vi "Delete me.vi"(10 "Debug":bool, 11 "State Pts in":T1) -> (2 "output cluster":cluster{dbl[], dbl[]}, 3 "State Pts out":T1)   [LabVIEW 2012]
uses:
  STARCO-Dev/RT-PID/support/P-h Diagram/States In.ctl
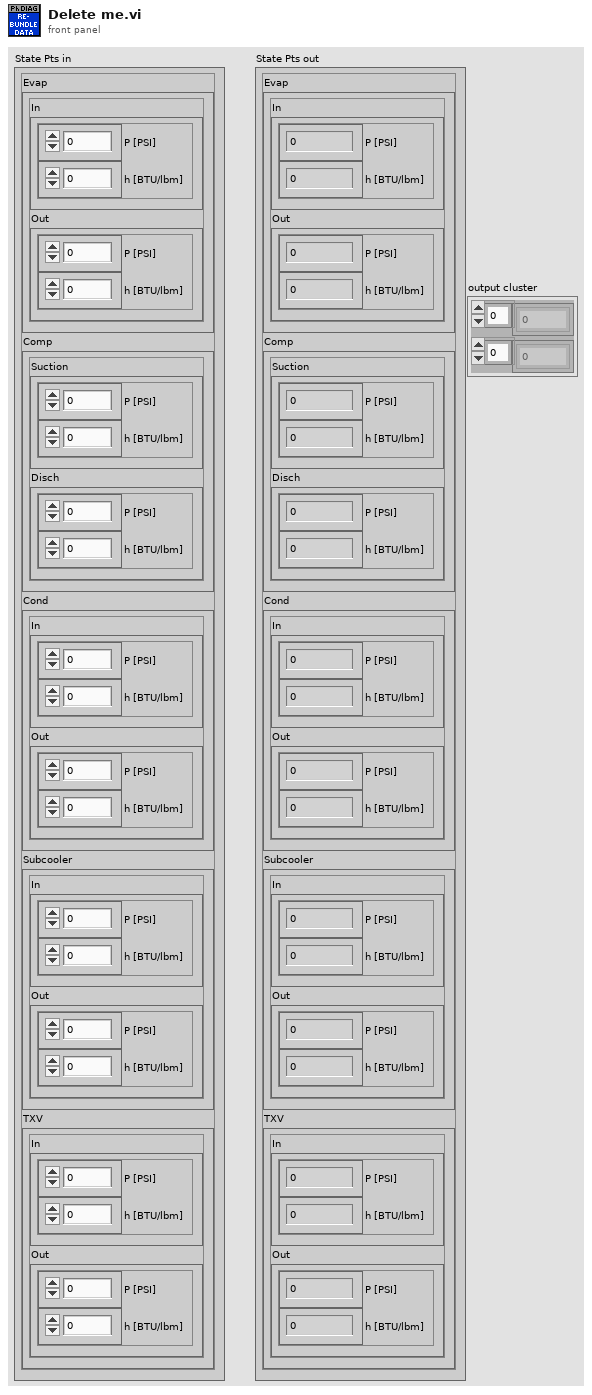
[diagram p1: front panel]
types:
  T1 = typedef "States In.ctl" = cluster{"Evap":cluster{"In":cluster{"P [PSI]":dbl, "h [BTU/lbm]":dbl}, "Out":cluster{"P [PSI]":dbl, "h [BTU/lbm]":dbl}}, "Comp":cluster{"Suction":cluster{"P [PSI]":dbl, "h [BTU/lbm]":dbl}, "Disch":cluster{"P [PSI]":dbl, "h [BTU/lbm]":dbl}}, "Cond":cluster{"In":cluster{"P [PSI]":dbl, "h [BTU/lbm]":dbl}, "Out":cluster{"P [PSI]":dbl, "h [BTU/lbm]":dbl}}, "Subcooler":cluster{"In":cluster{"P [PSI]":dbl, "h [BTU/lbm]":dbl}, "Out":cluster{"P [PSI]":dbl, "h [BTU/lbm]":dbl}}, "TXV":cluster{"In":cluster{"P [PSI]":dbl, "h [BTU/lbm]":dbl}, "Out":cluster{"P [PSI]":dbl, "h [BTU/lbm]":dbl}}}
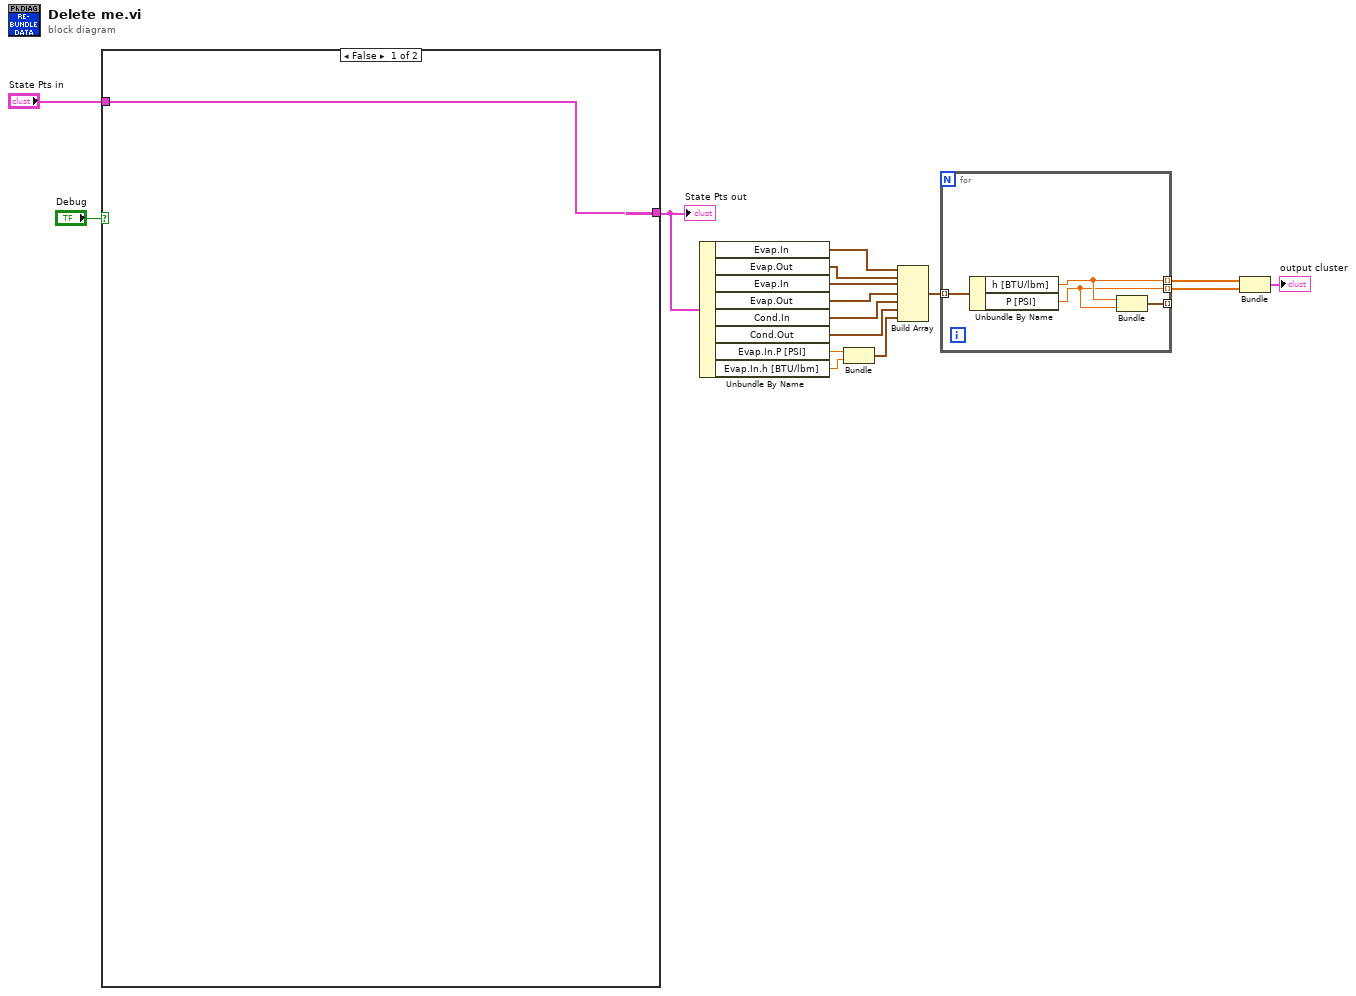
[diagram p0: block diagram]
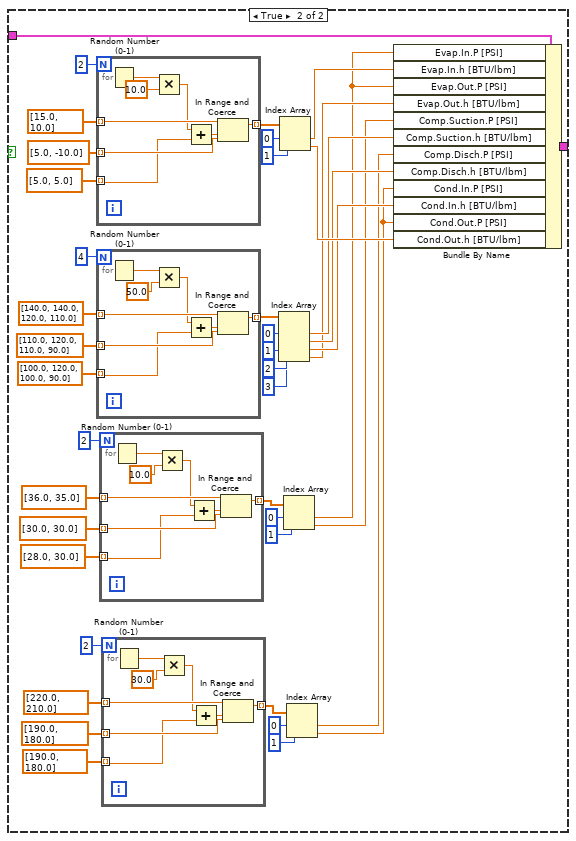
[diagram p2: hidden frame]
diagram:
  n1 = case shown="False" "Debug" {
    tunnel: "State Pts in" -> [w17 w59]
    tunnel: [w17 w58] -> w4
    frame False {
    }
    frame True {
      n2 = for {
        N: 2 -> [_]
        tunnel: dbl[] [15.0, 10.0] -> [w89] mode=indexing
        tunnel: dbl[] [5.0, -10.0] -> [w88] mode=indexing
        tunnel: dbl[] [5.0, 5.0] -> [w86] mode=indexing
        tunnel: [w85] -> w45 mode=indexing
        n3 = Random Number (0-1)() -> (number: 0 to 1=w90:dbl)
        n4 = Multiply(x=w90, y=10.0) -> (x*y=w87:dbl)
        n5 = Add(x=w87, y=w86) -> (x+y=w84:dbl)
        n6 = In Range and Coerce(upper limit=w89, x=w84, lower limit=w88) -> (coerced(x)=w85:dbl)  [unwired: 1 out]
      }
      n7 = for {
        N: 4 -> [_]
        tunnel: dbl[] [140.0, 140.0, 120.0, 110.0] -> [w81] mode=indexing
        tunnel: dbl[] [110.0, 120.0, 110.0, 90.0] -> [w80] mode=indexing
        tunnel: dbl[] [100.0, 120.0, 100.0, 90.0] -> [w78] mode=indexing
        tunnel: [w77] -> w38 mode=indexing
        n8 = Random Number (0-1)() -> (number: 0 to 1=w82:dbl)
        n9 = Multiply(x=w82, y=50.0) -> (x*y=w79:dbl)
        n10 = Add(x=w79, y=w78) -> (x+y=w76:dbl)
        n11 = In Range and Coerce(upper limit=w81, x=w76, lower limit=w80) -> (coerced(x)=w77:dbl)  [unwired: 1 out]
      }
      n12 = for {
        N: 2 -> [_]
        tunnel: dbl[] [36.0, 35.0] -> [w73] mode=indexing
        tunnel: dbl[] [30.0, 30.0] -> [w72] mode=indexing
        tunnel: dbl[] [28.0, 30.0] -> [w70] mode=indexing
        tunnel: [w69] -> w29 mode=indexing
        n13 = Random Number (0-1)() -> (number: 0 to 1=w74:dbl)
        n14 = Multiply(x=w74, y=10.0) -> (x*y=w71:dbl)
        n15 = Add(x=w71, y=w70) -> (x+y=w68:dbl)
        n16 = In Range and Coerce(upper limit=w73, x=w68, lower limit=w72) -> (coerced(x)=w69:dbl)  [unwired: 1 out]
      }
      n17 = for {
        N: 2 -> [_]
        tunnel: dbl[] [220.0, 210.0] -> [w65] mode=indexing
        tunnel: dbl[] [190.0, 180.0] -> [w64] mode=indexing
        tunnel: dbl[] [190.0, 180.0] -> [w62] mode=indexing
        tunnel: [w61] -> w21 mode=indexing
        n18 = Random Number (0-1)() -> (number: 0 to 1=w66:dbl)
        n19 = Multiply(x=w66, y=30.0) -> (x*y=w63:dbl)
        n20 = Add(x=w63, y=w62) -> (x+y=w60:dbl)
        n21 = In Range and Coerce(upper limit=w65, x=w60, lower limit=w64) -> (coerced(x)=w61:dbl)  [unwired: 1 out]
      }
      n22 = Index Array(array=w38, index #1=0 ("index"), index #2=1 ("index"), index #3=2 ("index"), index #4=3 ("index")) -> (element #1=w36:dbl, element #2=w34:dbl, element #3=w35:dbl, element #4=w32:dbl)
      n23 = Index Array(array=w45, index #1=0 ("index"), index #2=1 ("index")) -> (element #1=w42:dbl, element #2=w41:dbl)
      n24 = Index Array(array=w29, index #1=0 ("index"), index #2=1 ("index")) -> (element #1=w24:dbl, element #2=w18:dbl)
      n25 = Index Array(array=w21, index #1=0 ("index"), index #2=1 ("index")) -> (element #1=w20:dbl, element #2=w19:dbl)
      n26 = Bundle By Name(cluster=w59, "Evap.In.P [PSI]"=w24, "Evap.In.h [BTU/lbm]"=w42, "Evap.Out.P [PSI]"=w24, "Evap.Out.h [BTU/lbm]"=w32, "Comp.Suction.P [PSI]"=w18, "Comp.Suction.h [BTU/lbm]"=w36, "Comp.Disch.P [PSI]"=w20, "Comp.Disch.h [BTU/lbm]"=w34, "Cond.In.P [PSI]"=w19, "Cond.In.h [BTU/lbm]"=w35, "Cond.Out.P [PSI]"=w19, "Cond.Out.h [BTU/lbm]"=w41) -> (w58:T1)
    }
  }
  "State Pts out" <- w4
  n27 = Unbundle By Name(w4) -> ("Evap.In"=w13:cluster{"P [PSI]":dbl, "h [BTU/lbm]":dbl}, "Evap.Out"=w12:cluster{"P [PSI]":dbl, "h [BTU/lbm]":dbl}, "Evap.In"=w11:cluster{"P [PSI]":dbl, "h [BTU/lbm]":dbl}, "Evap.Out"=w10:cluster{"P [PSI]":dbl, "h [BTU/lbm]":dbl}, "Cond.In"=w9:cluster{"P [PSI]":dbl, "h [BTU/lbm]":dbl}, "Cond.Out"=w8:cluster{"P [PSI]":dbl, "h [BTU/lbm]":dbl}, "Evap.In.P [PSI]"=w14:dbl, "Evap.In.h [BTU/lbm]"=w6:dbl)
  n28 = Bundle("P [PSI]"=w14, "h [BTU/lbm]"=w6) -> (w5:cluster{"P [PSI]":dbl, "h [BTU/lbm]":dbl})  [unwired: 1 in]
  n29 = Build Array(w13, w12, w11, w10, w9, w8, w5) -> (w7:cluster{"P [PSI]":dbl, "h [BTU/lbm]":dbl}[])
  n30 = for {
    tunnel: [w94] -> w3 mode=indexing
    tunnel: [w93] -> w2 mode=indexing
    tunnel: w7 -> [w95] mode=indexing
    tunnel: [w92] -> _ mode=indexing
    n31 = Unbundle By Name(w95) -> ("h [BTU/lbm]"=w94:dbl, "P [PSI]"=w93:dbl)
    n32 = Bundle("h [BTU/lbm]"=w94, "P [PSI]"=w93) -> (w92:cluster{"h [BTU/lbm]":dbl, "P [PSI]":dbl})  [unwired: 1 in]
  }
  n33 = Bundle(w3, w2) -> (→"output cluster":cluster{dbl[], dbl[]})  [unwired: 1 in]
